vi "tdms testing.vi"() -> ()   [LabVIEW 2011]
panel:
  in  "Model_Number (FRED)":string="FRED"
  in  "Runs per File (5)":i32=5
  in  "Test Files (1)":i32=1
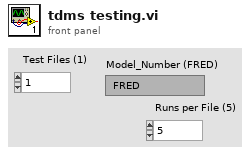
[diagram p1: front panel]
types:
  T1 = enum16{"open", "open or create", "create or replace", "create", "open (read-only)"}
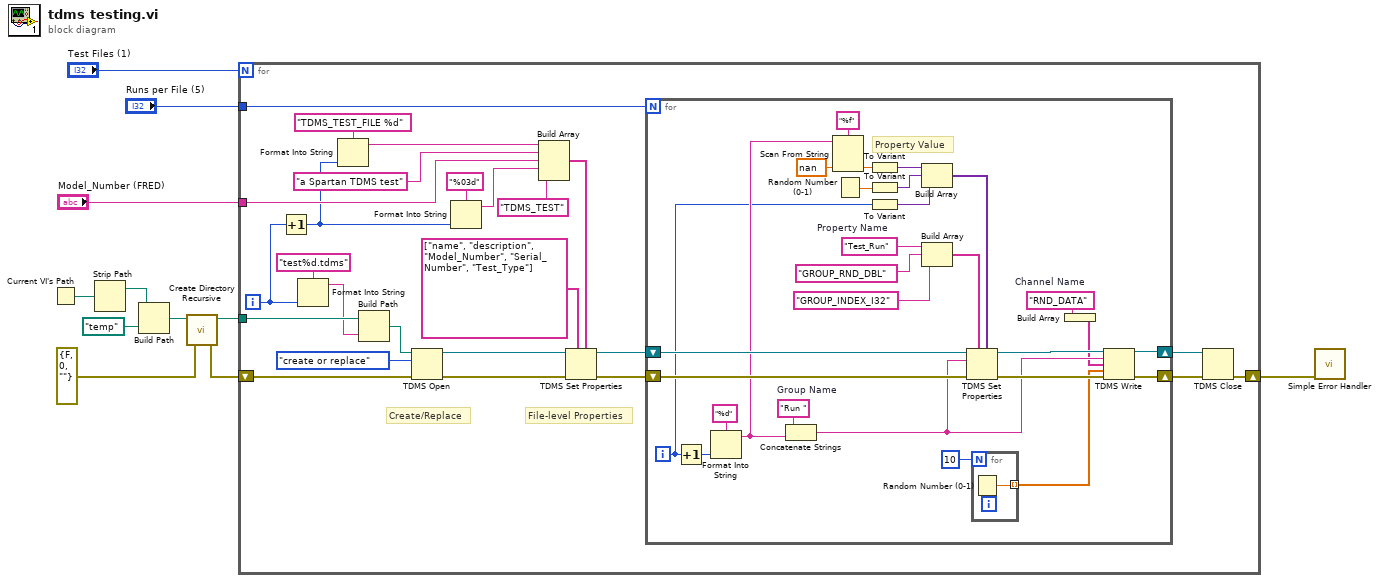
[diagram p0: block diagram]
diagram:
  n1 = Current VI's Path() -> (path=w11:path)
  n2 = Strip Path(path=w11) -> (stripped path=w10:path)  [unwired: 1 out]
  n3 = Build Path(base path=w10, name or relative path=path "temp") -> (appended path=w8:path)
  n4 = call <vilib>:"Create Directory Recursive.vi"("error in (no error)"=errorcluster {"status"=FALSE, "code"=0, "source"=""} ("error out"), "directory"=w8) -> ("error out"=w5:errorcluster, "directory copy"=w7:path)  [unwired: 1 in, 3 out]
  n5 = for {
    N: "Test Files (1)" -> [_]
    shift-right: [w22] -> w3
    shift-left: w5 -> [w28]
    tunnel: w7 -> [w26]
    tunnel: "Runs per File (5)" -> [w21]
    tunnel: "Model_Number (FRED)" -> [w16]
    i -> [w24]
    # "File-level Properties"
    # "Create/Replace"
    n6 = Increment(x=w24) -> (x+1=w12:i32)
    n7 = Format Into String(format string="test%d.tdms", w24) -> (resulting string=w23:string)  [unwired: 2 in, 1 out]
    n8 = Format Into String(format string="TDMS_TEST_FILE %d", w12) -> (resulting string=w35:string)  [unwired: 2 in, 1 out]
    n9 = Build Path(base path=w26, name or relative path=w23) -> (appended path=w27:path)
    n10 = TDMS Open(8:w28, 10:T1."create or replace" ("operation (0:open)"), 11:w27) -> (0:w33:errorcluster, 3:w32:refnum<k34>)  [unwired: 3 in]
    n11 = Format Into String(format string="%03d", w12) -> (resulting string=w14:string)  [unwired: 2 in, 1 out]
    n12 = Build Array(w35, "a Spartan TDMS test", w16, w14, "TDMS_TEST") -> (w30:string[])
    n13 = TDMS Set Properties(5:w30, 7:string[] ["name", "description", "Model_Number", "Serial_Number", "Test_Type"], 8:w33, 11:w32) -> (0:w20:errorcluster, 3:w18:refnum<k34>)  [unwired: 4 out]
    n14 = for {
      N: w21 -> [_]
      shift-right: [w43] -> w17
      shift-left: w18 -> [w56]
      shift-right: [w44] -> w19
      shift-left: w20 -> [w57]
      i -> [w47]
      w40 = "RND_DATA"  # Channel Name
      w52 = "Run "  # Group Name
      w61 = "Test_Run"  # Property Name
      # "Property Value"
      n15 = Increment(x=w47) -> (x+1=w54:i32)
      n16 = Format Into String(format string="%d", w54) -> (resulting string=w53:string)  [unwired: 2 in, 1 out]
      n17 = Concatenate Strings(w52, w53) -> (w42:string)
      n18 = Scan From String(format string="%f", input string=w53, default 1=nan) -> (output 1=w64:dbl)  [unwired: 2 in, 3 out]
      n19 = Random Number (0-1)() -> (number: 0 to 1=w49:dbl)
      n20 = To Variant(anything=w64) -> (Variant=w59:variant)
      n21 = To Variant(anything=w49) -> (Variant=w50:variant)
      n22 = To Variant(anything=w47) -> (Variant=w48:variant)
      n23 = Build Array(w59, w50, w48) -> (w58:variant[])
      n24 = Build Array(w61, "GROUP_RND_DBL", "GROUP_INDEX_I32") -> (w60:string[])
      n25 = TDMS Set Properties(5:w58, 7:w60, 8:w57, 10:w42, 11:w56) -> (0:w45:errorcluster, 3:w46:refnum<k34>)  [unwired: 3 out]
      n26 = for {
        N: 10 -> [_]
        tunnel: [w65] -> w38 mode=indexing
        n27 = Random Number (0-1)() -> (number: 0 to 1=w65:dbl)
      }
      n28 = Build Array(w40) -> (w39:string[])
      n29 = TDMS Write(0:w46, 5:w42, 7:w39, 9:w38, 11:w45) -> (4:w43:refnum<k34>, 15:w44:errorcluster)  [unwired: 1 in, 2 out]
    }
    n30 = TDMS Close(8:w19, 11:w17) -> (0:w22:errorcluster)  [unwired: 1 out]
  }
  n31 = call <vilib>:"Simple Error Handler.vi"("error in (no error)"=w3) -> ()  [unwired: 4 in, 5 out]
